vi "Remove Filters.vi"(8 "error in (no error)":errorcluster, 10 "Filter IDs":string[](array[string]), 11 "Bus Monitor in":refnum<class "Bus Monitor.lvclass">) -> (0 "error out":errorcluster, 3 "Bus Monitor out":refnum<class "Bus Monitor.lvclass">)   [LabVIEW 2020, in "BCI-1553 API.lvlib" / "Bus Monitor.lvclass"]
doc: "Removes a set of filters with matching IDs from this Bus Monitor."
uses:
  Bus Monitor.lvclass
  Bus Monitor.lvclass/Bus Monitor.ctl
  Dependencies/Registry/Registry.lvclass/Registry.ctl
  Dependencies/Registry/Registry.lvclass
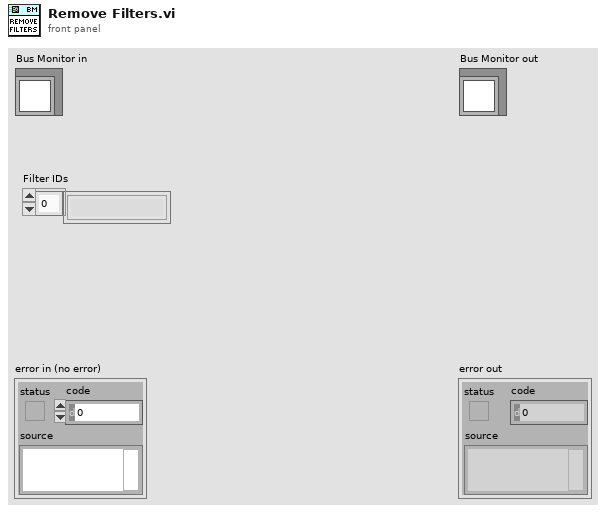
[diagram p1: front panel]
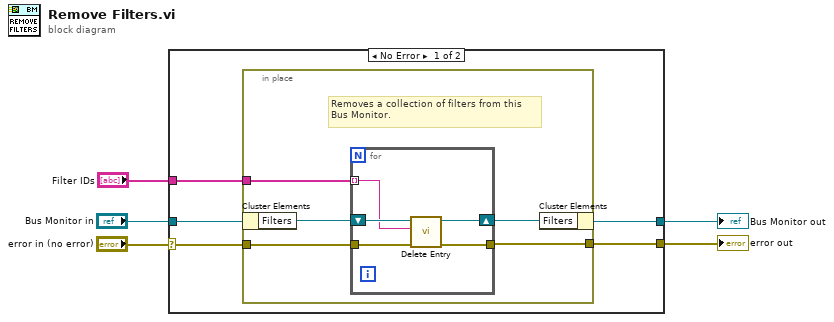
[diagram p0: block diagram]
diagram:
  n1 = case shown="No Error" "error in (no error)" {
    selector: "error in (no error)" -> [w7 w22]
    tunnel: [w8 w22] -> w1
    tunnel: [w9 w21] -> w2
    tunnel: "Bus Monitor in" -> [w10 w21]
    tunnel: "Filter IDs" -> [w6 _]
    frame No Error {
      n2 = in-place {
        in-place-border: [w12] -> w8
        in-place-border: w7 -> [w14]
        in-place-border: w6 -> [w11]
        # "Removes a collection of filters from this\nBus Monitor."
        n3 = in-place-cluster #1(w10) -> ("Filters"=w15:refnum<class "Registry.lvclass">)
        n4 = for {
          shift-right: [w17] -> w13
          shift-left: w15 -> [w20]
          tunnel: w14 -> [w19]
          tunnel: w11 -> [w18] mode=indexing
          tunnel: [w16] -> w12
          n5 = call "Delete Entry.vi"("error in (no error)"=w19, "Key"=w18, "Registry in"=w20) -> ("error out"=w16:errorcluster, "Registry out"=w17:refnum<class "Registry.lvclass">)  [unwired: 6 in, 1 out]
        }
        n6 = in-place-cluster #1("Filters"=w13) -> (w9:refnum<class "Bus Monitor.lvclass">)
      }
    }
    frame Error {
    }
  }
  "error out" <- w1
  "Bus Monitor out" <- w2
